vi "Control Calibration Board Relays.vi"(5 "Device Name":string="Dev1", 8 "error in":errorcluster, 9 "Resistance":T2, 10 "Channels":T1, 11 "Mode":T3) -> (0 "error out":errorcluster={"status"=TRUE, "code"=-200220, "source"="DAQmx Create Channel (DO-Digital Output).vi:2<append>\n<B>Device Specified: </B>Dev1\n\n<B>Task Name: </B>_unnamedTask<0>"})   [LabVIEW 2015]
uses:
  Relay Modes.ctl
  Resistances.ctl
  Channels_v2.ctl
panel:
  out "Array":cluster{bool, string}[](array[cluster])
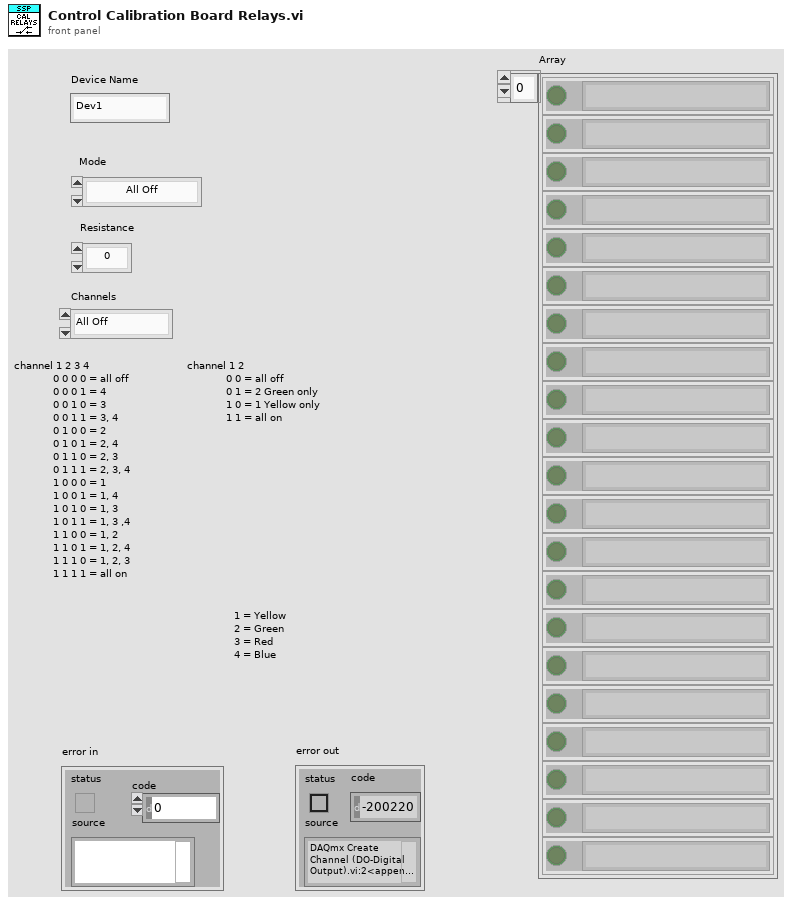
[diagram p1: front panel]
types:
  T1 = typedef "Channels_v2.ctl" = enum16{"All Off", "Channel 4", "Channel 3", "4,3", "Channel 2", "4,2", "3,2", "4,3,2,", "Channel 1", "4,1", "3,1", "4,3,1", "2,1", "4,2,1", "3,2,1", "All On"}
  T2 = typedef "Resistances.ctl" = enum16{"0", "20", "40", "200", "400", "2k", "4K", "20k", "40K", "200k", "400K", "2M", "4M"}
  T3 = typedef "Relay Modes.ctl" = enum16{"All Off", "Short", "Ohms", "Fluke", "Daq AO 0"}
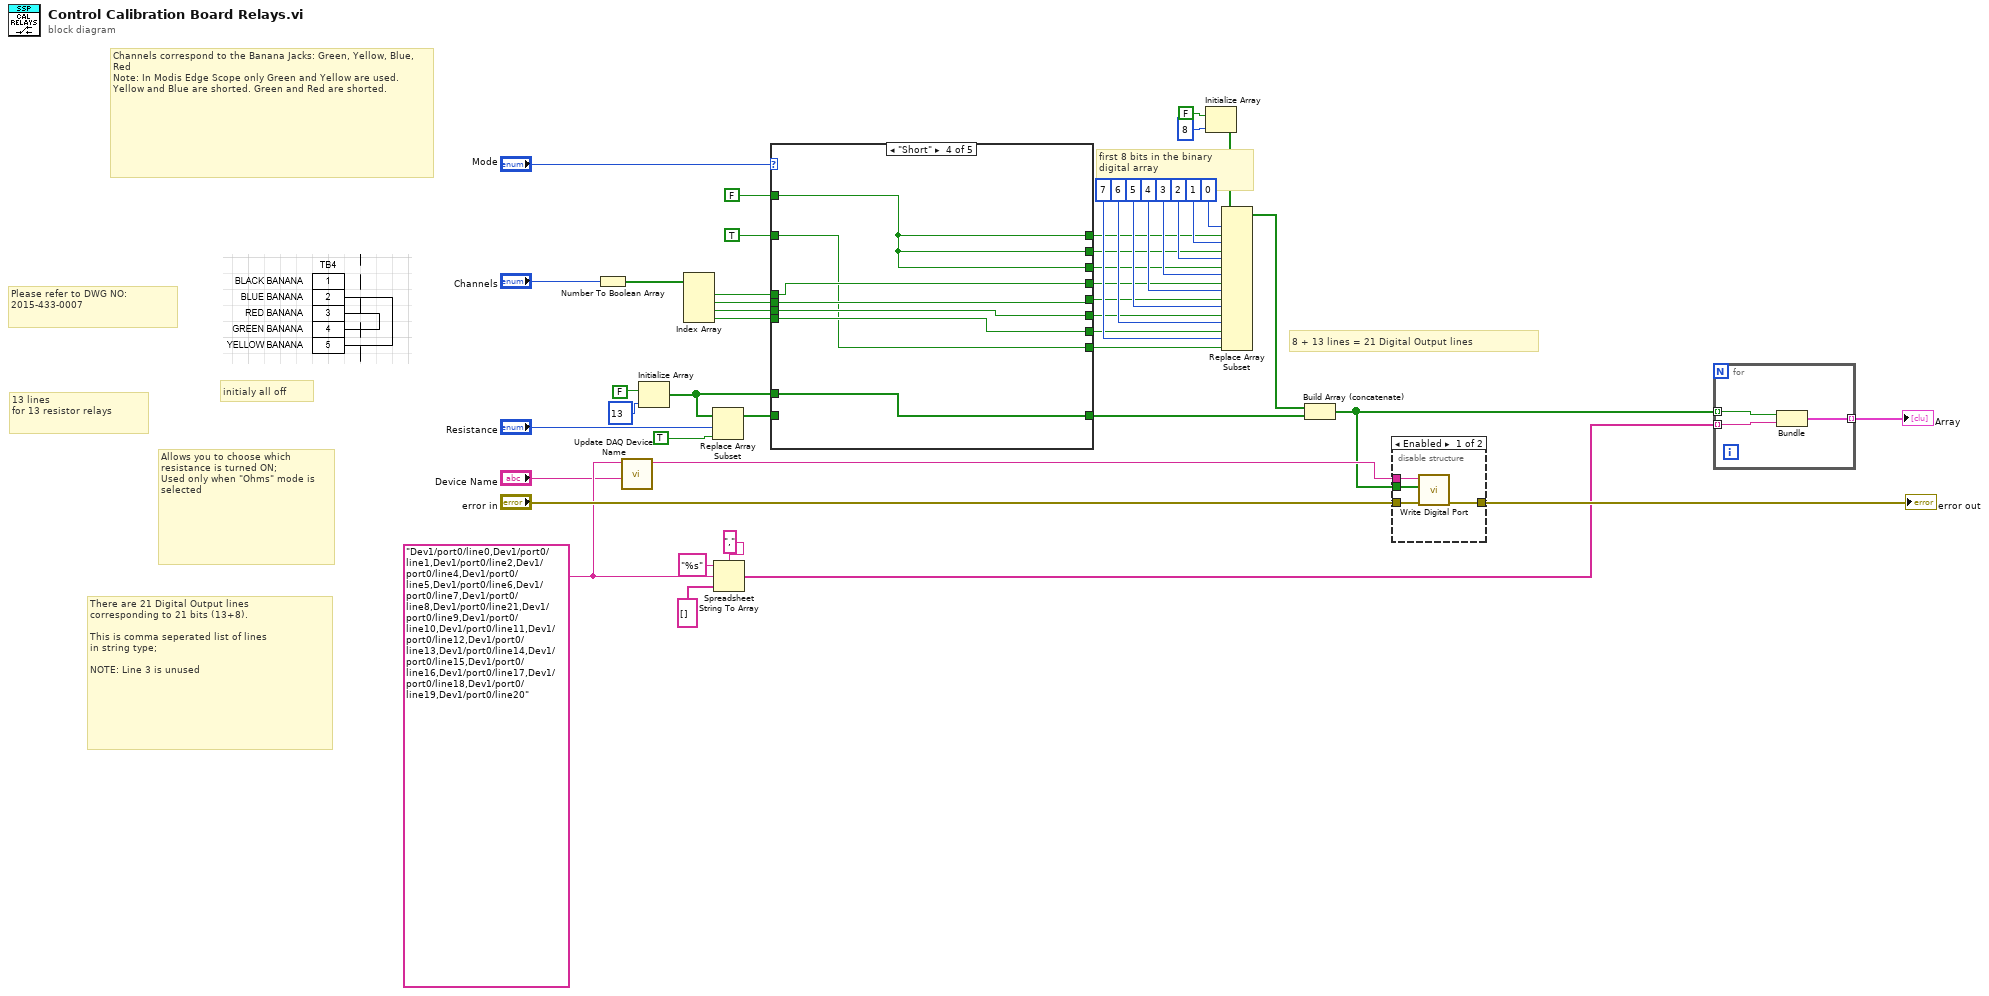
[diagram p0: block diagram]
diagram:
  w6 = "Dev1/port0/line0,Dev1/port0/line1,Dev1/port0/line2,Dev1/port0/line4,Dev1/port0/line5,Dev1/port0/line6,Dev1/port0/line7,Dev1/port0/line8,Dev1/port0/line21,Dev1/port0/line9,Dev1/port0/line10,Dev1/port0/line11,Dev1/port0/line12,Dev1/port0/line13,Dev1/port0/line14,Dev1/port0/line15,Dev1/port0/line16,Dev1/port0/line17,Dev1/port0/line18,Dev1/port0/line19,Dev1/port0/line20" ("String")
  # "Please refer to DWG NO:\n2015-433-0007"
  # "Allows you to choose which resistance is turned ON;\nUsed only when \"Ohms\" mode is selected"
  # "initialy all off"
  # "first 8 bits in the binary\ndigital array"
  # "Channels correspond to the Banana Jacks: Green, Yellow, Blue, Red\nNote: In Modis Edge Scope only Green and Yellow are used.\nYellow and Blue are shorted. Green and Red are shorted."
  # "13 lines\nfor 13 resistor relays"
  # "8 + 13 lines = 21 Digital Output lines"
  # "There are 21 Digital Output lines \ncorresponding to 21 bits (13+8).\n\nThis is comma seperated list of lines\nin string type;\n\nNOTE: Line 3 is unused"
  n1 = Number To Boolean Array(number="Channels") -> (Boolean array=w21:bool[])
  n2 = call "Update DAQ Device Name.vi"("Device Name"="Device Name", "Lines in (String)"=w6) -> ("Lines out (DAQmx Physical Channels)"=w16:tag)  [unwired: 9 in]
  n3 = Initialize Array(FALSE, 13 ("dimension size")) -> (w27:bool[])
  n4 = Index Array(array=w21) -> (element #1=w20:bool, element #2=w19:bool, element #3=w18:bool, element #4=w17:bool)  [unwired: 4 in]
  n5 = Replace Array Subset(array=w27, new element=TRUE, index="Resistance") -> (w29:bool[])
  n6 = Spreadsheet String To Array(delimiter (Tab)=",", format string="%s", spreadsheet string=w6, array type (2D Dbl)=string[] []) -> (array=w2:string[])
  n7 = case shown="\"Short\"" "Mode" {
    tunnel: w29 -> [_ w51 _ _ _]
    tunnel: [w49 w51 w58 w65 w72] -> w28
    tunnel: w27 -> [w49 _ w58 w65 w72]
    tunnel: FALSE -> [w48 w50 w52 w60 w68]
    tunnel: [w48 w50 w57 w60 w68] -> w25
    tunnel: TRUE -> [_ _ w57 w59 w71]
    tunnel: [w48 w50 w57 w60 w68] -> w23
    tunnel: [w48 w50 w52 w60 w71] -> w22
    tunnel: w20 -> [_ _ w56 w64 w67]
    tunnel: w19 -> [_ _ w55 w63 w70]
    tunnel: [w48 w50 w56 w64 w67] -> w15
    tunnel: [w48 w50 w55 w63 w70] -> w14
    tunnel: [w48 w50 w54 w62 w66] -> w13
    tunnel: w18 -> [_ _ w54 w62 w66]
    tunnel: w17 -> [_ _ w53 w61 w69]
    tunnel: [w48 w50 w53 w61 w69] -> w12
    tunnel: [w48 w50 w52 w59 w68] -> w11
    frame "All Off", Default {
      # "set all bits to False"
    }
    frame "Ohms" {
      # "in Ohms Mode, the first 8 bits\nare all set to False"
      # "Note that only \"Ohms\" option uses this\narray subset"
    }
    frame "Fluke" {
      # "in Fluke Mode, Resistance is unused"
    }
    frame "Short" {
    }
    frame "Daq AO 0" {
    }
  }
  n8 = Initialize Array(FALSE, 8 ("dimension size")) -> (w45:bool[])
  n9 = Replace Array Subset(array=w45, new element #1=w25, index #1=0 ("index"), new element #2=w23, index #2=1 ("index"), new element #3=w22, index #3=2 ("index"), new element #4=w15, index #4=3 ("index"), new element #5=w14, index #5=4 ("index"), new element #6=w13, index #6=5 ("index"), new element #7=w12, index #7=6 ("index"), new element #8=w11, index #8=7 ("index")) -> (w7:bool[])
  n10 = Build Array (concatenate)(w7, w28) -> (w3:bool[])
  n11 = disable-structure shown="Enabled" {
    disable-tunnel: "error in" -> [w76 _]
    disable-tunnel: [w75 _] -> w34
    disable-tunnel: w3 -> [w74 _]
    disable-tunnel: w16 -> [w73 _]
    frame Enabled {
      n12 = call "Write Digital Port.vi"("error in"=w76, "Data"=w74, "Line(s)"=w73) -> ("error out"=w75:errorcluster)  [unwired: 8 in]
    }
    frame Disabled {
    }
  }
  "error out" <- w34
  n13 = for {
    tunnel: w3 -> [w79] mode=indexing
    tunnel: w2 -> [w78] mode=indexing
    tunnel: [w77] -> w1 mode=indexing
    n14 = Bundle(w79, w78) -> (w77:cluster{bool, string})  [unwired: 1 in]
  }
  "Array" <- w1
